vi "Vertical coords to select row.vi"(9 "Constant Sizes":T1, 10 "Coords.Vertical":i32, 11 "Tree.Position:Top":i32) -> (2 "Pixels from top of row":i32, 3 "Displayed Row":i32)   [LabVIEW 2020, in "BetterDragAndDrop.lvlib"]
uses:
  BetterDragAndDrop.lvlib
  Classes/BetterHandle/Pixel Constants.ctl
  Classes/BetterHandle/BetterHandle.lvclass
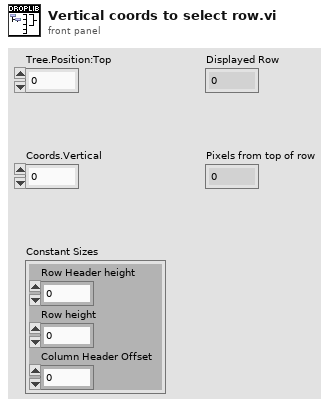
[diagram p1: front panel]
types:
  T1 = typedef "BetterDragAndDrop.lvlib/BetterHandle.lvclass/Pixel Constants.ctl" = cluster{"Row Header height":i32, "Row height":i32, "Column Header Offset":i32}
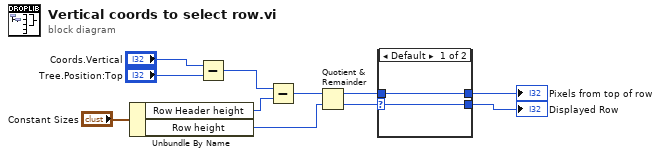
[diagram p0: block diagram]
diagram:
  n1 = Unbundle By Name("Constant Sizes") -> ("Row Header height"=w1:i32, "Row height"=w2:i32)
  n2 = Subtract(x="Coords.Vertical", y="Tree.Position:Top") -> (x-y=w11:i32)
  n3 = Subtract(x=w11, y=w1) -> (x-y=w10:i32)
  n4 = Quotient & Remainder(x=w10, y=w2) -> (x-y*floor(x/y)=w8:i32, floor(x/y)=w9:i32)
  n5 = case shown="Default" w9 {
    selector: w9 -> [w13 _]
    tunnel: w8 -> [w12 _]
    tunnel: [w13 _] -> w5
    tunnel: [w12 _] -> w4
    frame Default {
    }
    frame ..-1 {
    }
  }
  "Displayed Row" <- w5
  "Pixels from top of row" <- w4
